vi "WFDC Get CC Image.vi"(0 "Ref Images":T1[](array[typedef]), 2 "Half Shift":i32=7, 5 "Current Image":u16[][](array[numeric]), 11 "Error In":errorcluster) -> (8 "CC Image":dbl[][](array[numeric]), 15 "Error Out":errorcluster)   [LabVIEW 2020]
uses:
  <vilib>/vision/Image Controls.llb/IMAQ Image.ctl
  WFDC DLL and Testing/Visual Studio NCC Max Shift DLL/x64/Release/VSmaxShiftNCC.dll
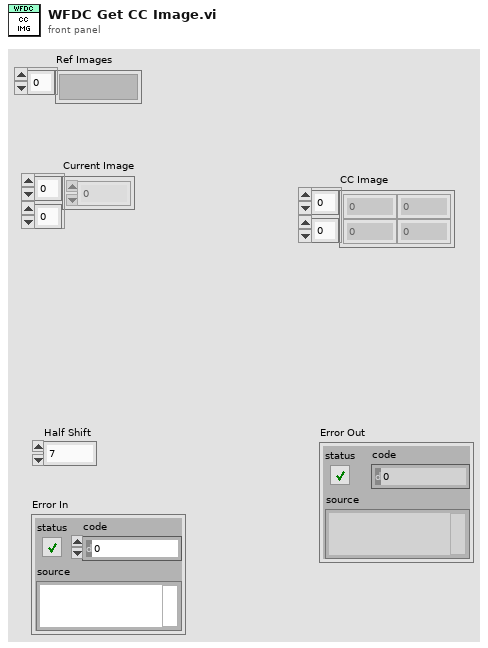
[diagram p1: front panel]
types:
  T1 = typedef "IMAQ Image.ctl" = refnum<image>
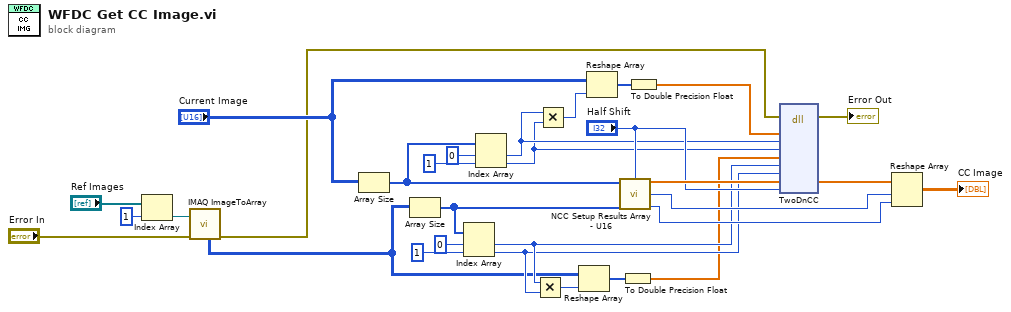
[diagram p0: block diagram]
diagram:
  n1 = Index Array(array="Ref Images", index=1) -> (element=w4:T1)
  n2 = call "IMAQ ImageToArray"("error in (no error)"="Error In", "Image"=w4) -> ("Image Pixels (U16)"=w3:u16[][], "error out"=w28:errorcluster)  [unwired: 2 in, 3 out]
  n3 = Array Size(array="Current Image") -> (size(s)=w12:i32[])
  n4 = Array Size(array=w3) -> (size(s)=w22:i32[])
  n5 = Index Array(array=w22, index #1=0 ("index"), index #2=1 ("index")) -> (element #1=w19:i32, element #2=w18:i32)
  n6 = Index Array(array=w12, index #1=0 ("index"), index #2=1 ("index")) -> (element #1=w9:i32, element #2=w8:i32)
  n7 = Multiply(x=w19, y=w18) -> (x*y=w17:i32)
  n8 = Multiply(x=w9, y=w8) -> (x*y=w7:i32)
  n9 = Reshape Array(w3, w17) -> (w16:u16[])
  n10 = Reshape Array("Current Image", w7) -> (w11:u16[])
  n11 = call "NCC Setup Results Array - U16.vi"("Image 01 Size"=w12, "Half Shift"="Half Shift", "Image 02 Size"=w22) -> ("NCC Results Array"=w27:dbl[], "Result Rows"=w24:i32, "Result Columns"=w25:i32)  [unwired: 10 in]
  n12 = To Double Precision Float(number=w16) -> (double precision float=w15:dbl[])
  n13 = To Double Precision Float(number=w11) -> (double precision float=w10:dbl[])
  n14 = dll-call lib="C:/Users/George Sirinakis/Documents/Microscope-Control/Microscope Modules/Wide Field Drift Correction/WFDC DLL and Testing/Visual Studio NCC Max Shift DLL/x64/Release/VSmaxShiftNCC.dll" fn="TwoDnCC"(error in=w28, "im01"=w10, "im01rowSize"=w9, "im01colSize"=w8, "im02"=w15, "im02rowSize"=w19, "im02ColSize"=w18, "theResult"=w27, "halfShift"="Half Shift") -> (error out=→"Error Out":errorcluster, "theResult"=w26:dbl[])  [unwired: 10 in, 1 out]
  n15 = Reshape Array(w26, w24, w25) -> (→"CC Image":dbl[][])
